vi "test_BigDataFits_U16_FGV.vi"() -> ()   [LabVIEW 2020]
uses:
  ClustBigFilFits.ctl
  DataTyp_Header.ctl
  BigDataFits.ctl
panel:
  out "sortie d'erreur":errorcluster
  in  "ClustBigFilFits":T1={"file (use dialog)"=path "D:/DATA/Imatest.fits", "Type de données"=enum."I16 (signed integer 16bit)", "Commentaire"="", "naxis1"=0, "naxis2"=0, "naxis3"=1, "Exptime"=1.0}
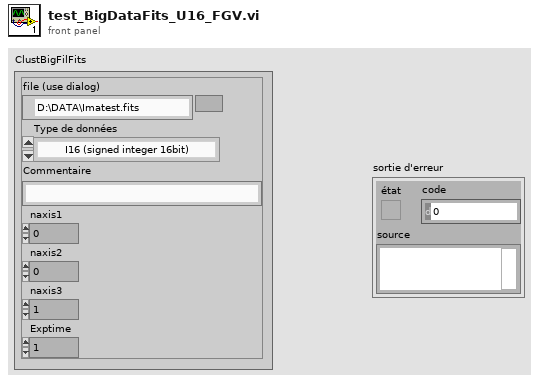
[diagram p1: front panel]
types:
  T1 = typedef "ClustBigFilFits.ctl" = cluster{"file (use dialog)":path, "Type de données":T2, "Commentaire":string, "naxis1":i32, "naxis2":i32, "naxis3":i32, "Exptime":sgl}
  T2 = typedef "DataTyp_Header.ctl" = enum16{"U8 (unsigned integer 8bit)", "I16 (signed integer 16bit)", "U16 (unsigned integer 16 bit)", "I32 (signed integer 32bit)", "U32 (unsigned integer 32 bit)", "SGL (float 32bit)", "DBL(float 64bit)", "complex (2xfloat 64bit)"}
  T3 = typedef "BigDataFits.ctl" = enum16{"Init", "WritHeader", "WritData", "Close"}
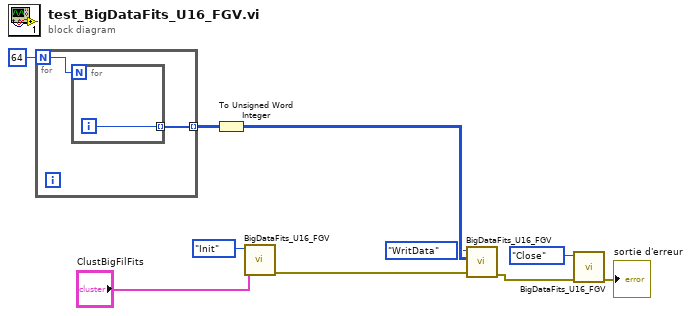
[diagram p0: block diagram]
diagram:
  n1 = for {
    N: 64 -> [w12]
    tunnel: [w11] -> w8 mode=indexing
    n2 = for {
      N: w12 -> [_]
      tunnel: [w13] -> w11 mode=indexing
      i -> [w13]
    }
  }
  n3 = To Unsigned Word Integer(number=w8) -> (unsigned 16bit integer=w7:u16[][])
  n4 = call "BigDataFits_U16_FGV.vi"("ClustBigFilFits"="ClustBigFilFits", "Énum"=BigDataFits."Init") -> ("sortie d'erreur"=w6:errorcluster)  [unwired: 9 in]
  n5 = call "BigDataFits_U16_FGV.vi"("InError"=w6, "entier 16 bits"=w7, "Énum"=BigDataFits."WritData") -> ("sortie d'erreur"=w9:errorcluster)  [unwired: 8 in]
  n6 = call "BigDataFits_U16_FGV.vi"("InError"=w9, "Énum"=BigDataFits."Close") -> ("sortie d'erreur"=→"sortie d'erreur":errorcluster)  [unwired: 9 in]
